vi "Controller - State Exit.vi"(8 "error in (no error)":errorcluster, 11 "View Model":T1) -> (0 "error out":errorcluster, 3 "View Model":T1)   [LabVIEW 2017]
doc: "Process state during car wash step/cycle completion."
uses:
  View Model/Controls/View Model.ctl
  View Model/Controls/Shared Model.ctl
  Error Handler/Controls/Error Model.ctl
  Error Handler/Controls/Error Data.ctl
  Error Handler/Controls/Error Level.ctl
  Configuration/Controls/Config Model.ctl
  Configuration/Controls/Config Record.ctl
  Configuration/Controls/Config Data.ctl
  Configuration/Controls/Config Command.ctl
  Controls/Controler Model.ctl
  Views/Vehicle Position View/Controls/Vehicle - Station Slider.ctl
  Views/Entry Console View/Controls/Entry Console - Wash Steps.ctl
  Controls/Controller - Event.ctl
  Controls/Controller - Commands.ctl
  Controls/Controller - Overhead.ctl
  Controls/Controller - States.ctl
  Controls/Controller - Wash Step.ctl
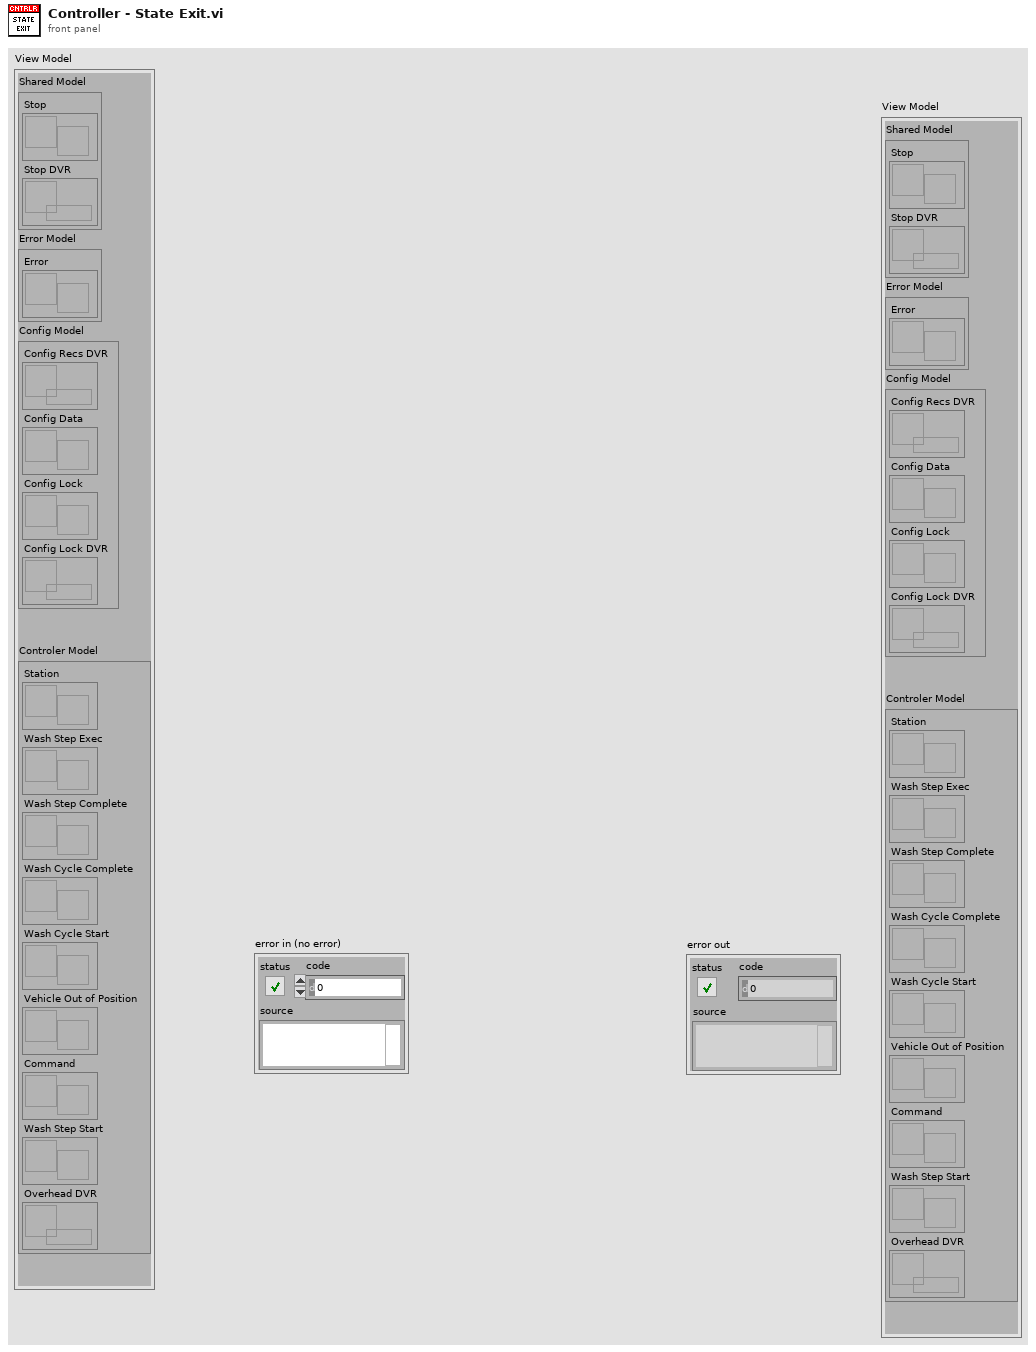
[diagram p1: front panel]
types:
  T1 = typedef "View Model.ctl" = cluster{"Shared Model":T2, "Error Model":T3, "Config Model":T4, "Controler Model":T5}
  T2 = typedef "Shared Model.ctl" = cluster{"Stop":refnum<user-event>, "Stop DVR":refnum<data-value>}
  T3 = typedef "Error Model.ctl" = cluster{"Error":refnum<user-event>}
  T4 = typedef "Config Model.ctl" = cluster{"Config Recs DVR":refnum<data-value>, "Config Data":refnum<user-event>, "Config Lock":refnum<user-event>, "Config Lock DVR":refnum<data-value>}
  T5 = typedef "Controler Model.ctl" = cluster{"Station":refnum<user-event>, "Wash Step Exec":refnum<user-event>, "Wash Step Complete":refnum<user-event>, "Wash Cycle Complete":refnum<user-event>, "Wash Cycle Start":refnum<user-event>, "Vehicle Out of Position":refnum<user-event>, "Command":refnum<user-event>, "Wash Step Start":refnum<user-event>, "Overhead DVR":refnum<data-value>}
  T6 = typedef "Controller - States.ctl" = enum16{"Initial", "Wait for Start", "Wash Cycle Start", "Wait for Vehicle Position", "Wash Step Start", "Wash Step Execute", "Wash Step Complete", "Wash Cycle Complete", "Wash Exit", "Wash Abort/Terminate"}
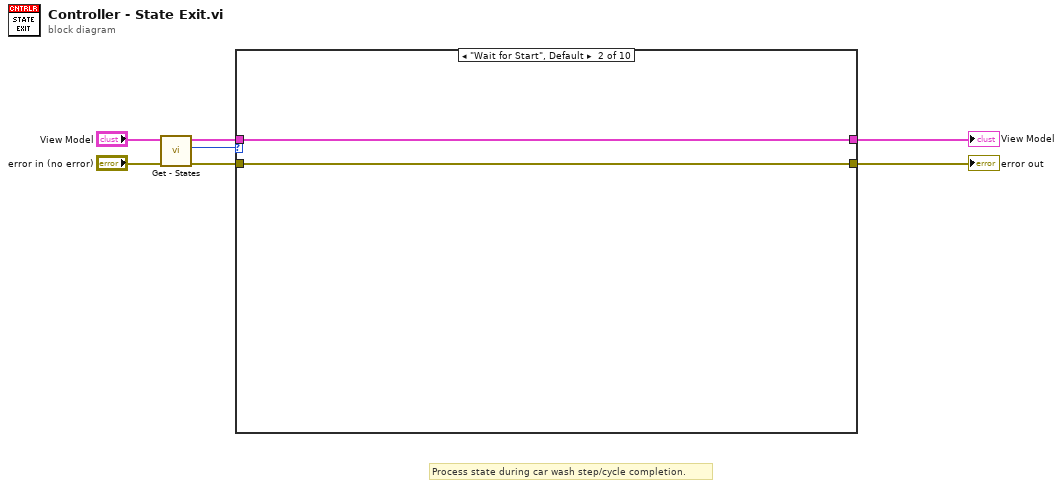
[diagram p0: block diagram]
diagram:
  # "Process state during car wash step/cycle completion."
  n1 = call "Get - States.vi"("error in (no error)"="error in (no error)", "View Model"="View Model") -> ("error out"=w3:errorcluster, "Current State"=w5:T6, "View Model"=w4:T1)  [unwired: 6 in, 1 out]
  n2 = case shown="\"Wait for Start\", Default" w5 {
    tunnel: w4 -> [w9 w11 w13 w15 w17 w19 w21 w23 w25 w27]
    tunnel: w3 -> [w8 w10 w12 w14 w16 w18 w20 w22 w24 w26]
    tunnel: [w9 w11 w13 w15 w17 w19 w21 w23 w25 w27] -> w1
    tunnel: [w8 w10 w12 w14 w16 w18 w20 w22 w24 w26] -> w2
    frame "Initial" {
    }
    frame "Wait for Start", Default {
    }
    frame "Wash Cycle Start" {
    }
    frame "Wait for Vehicle Position" {
    }
    frame "Wash Step Start" {
    }
    frame "Wash Step Execute" {
    }
    frame "Wash Step Complete" {
    }
    frame "Wash Cycle Complete" {
    }
    frame "Wash Exit" {
    }
    frame "Wash Abort/Terminate" {
    }
  }
  "error out" <- w2
  "View Model" <- w1
